vi "Register Events.vi"(8 "Error In":errorcluster, 11 "WebView in":refnum<class "WebView.lvclass">) -> (0 "Error Out":errorcluster, 2 "Events":T1, 3 "WebView out":refnum<class "WebView.lvclass">)   [LabVIEW 2024, in "WebView.lvclass"]
uses:
  WebView.lvclass
  Events--cluster.ctl
  Navigation Complete Event Data--cluster.ctl
  Source Changed Event Data--cluster.ctl
  Navigation Start Event Data--cluster.ctl
  <vilib>/sklein/WebView2/Libs/Microsoft.Web.WebView2.Core.dll
  WebView.lvclass/WebView.ctl
  callbacks/Raise Navigation Complete Event.vi
  callbacks/Raise Navigation Starting Event.vi
  callbacks/Raise Source Changed Event.vi
  callbacks/Raise Document Title Changed Event.vi
  callbacks/Raise Status Bar Text Changed Event.vi
  callbacks/Raise WebMessage Received Event.vi
  callbacks/Raise Window Close Requested Event.vi
  callbacks/Raise Dom Content Loaded Event.vi
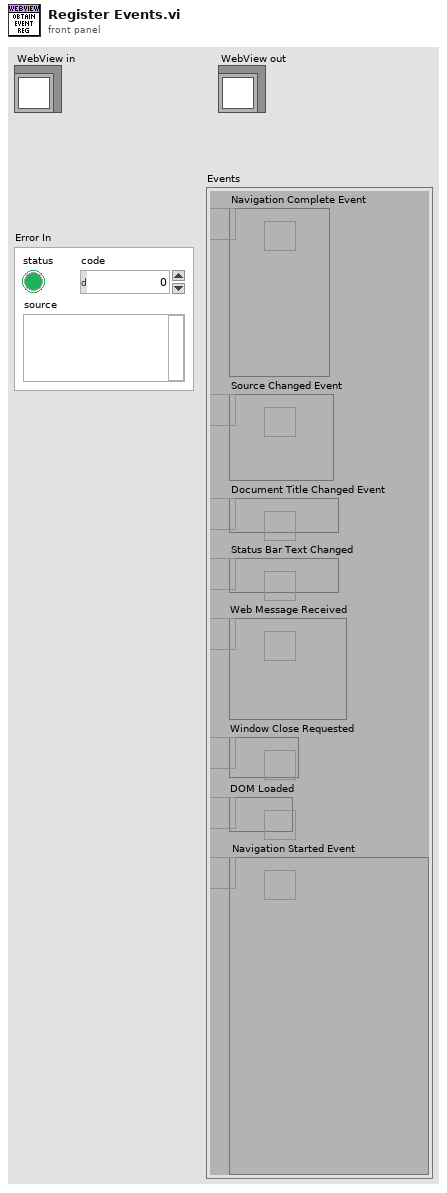
[diagram p1: front panel]
types:
  T1 = typedef "WebView.lvclass/Events--cluster.ctl" = cluster{"Navigation Complete Event":refnum<user-event>, "Source Changed Event":refnum<user-event>, "Document Title Changed Event":refnum<user-event>, "Status Bar Text Changed":refnum<user-event>, "Web Message Received":refnum<user-event>, "Window Close Requested":refnum<user-event>, "DOM Loaded":refnum<user-event>, "Navigation Started Event":refnum<user-event>}
  T2 = typedef "WebView.lvclass/Resources--cluster.ctl" = cluster{"WebView2 Control":refnum<k24>, "Webview2 Core":refnum<k24>, "event callback":refnum<k27>, "Environment":refnum<k24>}
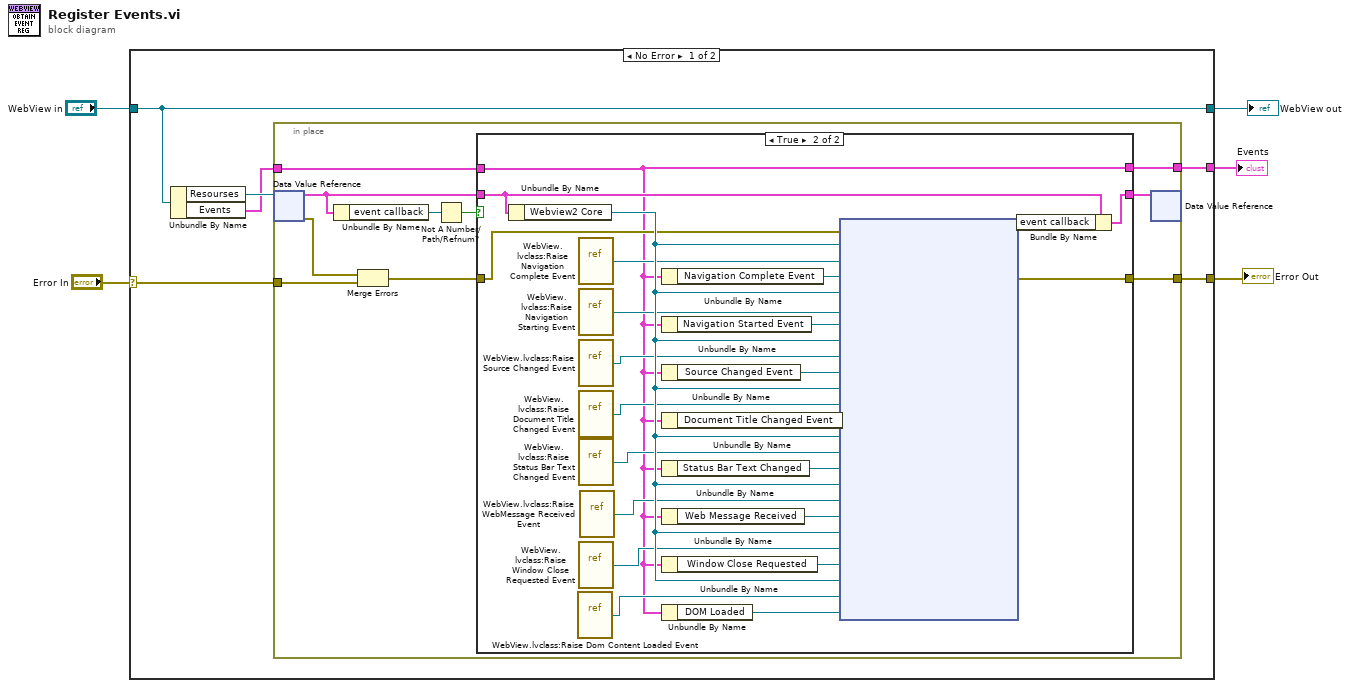
[diagram p0: block diagram]
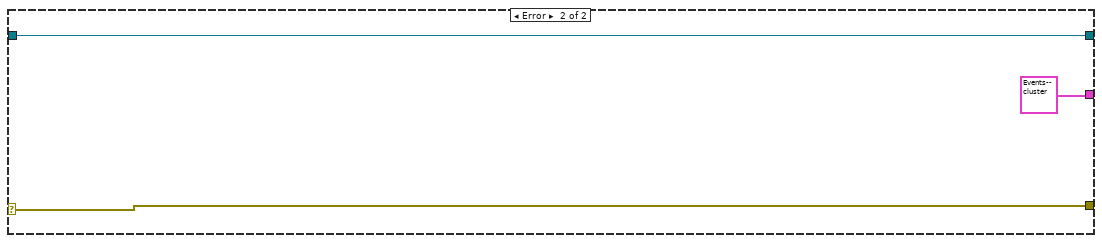
[diagram p3: hidden frame]
diagram:
  n1 = case shown="No Error" "Error In" {
    selector: "Error In" -> [w9 w50]
    tunnel: [w8 w50] -> w4
    tunnel: [w11 w49] -> w2
    tunnel: "WebView in" -> [w11 w49]
    tunnel: [w6 T1 {"Navigation Complete Event"=refnum, "Source Changed Event"=refnum, "Document Title Changed Event"=refnum, "Status Bar Text Changed"=refnum, "Web Message Received"=refnum, "Window Close Requested"=refnum, "DOM Loaded"=refnum, "Navigation Started Event"=refnum} ("Events")] -> w1
    frame No Error {
      n2 = Unbundle By Name(w11) -> ("Resourses"=w10:refnum<data-value>, "Events"=w7:T1)
      n3 = in-place {
        in-place-border: w9 -> [w21]
        in-place-border: [w18] -> w8
        in-place-border: w7 -> [w13]
        in-place-border: [w12] -> w6
        n4 = in-place-dvr #1(w10) -> (w15:T2, w20:errorcluster)
        n5 = Unbundle By Name(w15) -> ("event callback"=w17:refnum<k27>)
        n6 = Merge Errors(w20, w21) -> (w19:errorcluster)
        n7 = Not A Number/Path/Refnum?(number/path/refnum=w17) -> (NaN/Path/Refnum?=w16:bool)
        n8 = case shown="True" w16 {
          tunnel: [w24 w47] -> w18
          tunnel: w19 -> [w24 w42]
          tunnel: w15 -> [w23 w44]
          tunnel: [w23 w45] -> w14
          tunnel: w13 -> [w22 w33]
          tunnel: [w22 w33] -> w12
          frame False {
          }
          frame True {
            n9 = Unbundle By Name(w44) -> ("Webview2 Core"=w43:refnum<k24>)
            n10 = vi-ref "WebView.lvclass:Raise Dom Content Loaded Event.vi"() -> (w34:refnum<vi>)
            n11 = vi-ref "WebView.lvclass:Raise Navigation Complete Event.vi"() -> (w41:refnum<vi>)
            n12 = vi-ref "WebView.lvclass:Raise Navigation Starting Event.vi"() -> (w40:refnum<vi>)
            n13 = vi-ref "WebView.lvclass:Raise Source Changed Event.vi"() -> (w39:refnum<vi>)
            n14 = vi-ref "WebView.lvclass:Raise Document Title Changed Event.vi"() -> (w38:refnum<vi>)
            n15 = vi-ref "WebView.lvclass:Raise Status Bar Text Changed Event.vi"() -> (w37:refnum<vi>)
            n16 = vi-ref "WebView.lvclass:Raise Window Close Requested Event.vi"() -> (w35:refnum<vi>)
            n17 = vi-ref "WebView.lvclass:Raise WebMessage Received Event.vi"() -> (w36:refnum<vi>)
            n18 = Unbundle By Name(w33) -> ("Navigation Complete Event"=w32:refnum<user-event>)
            n19 = Unbundle By Name(w33) -> ("Navigation Started Event"=w31:refnum<user-event>)
            n20 = Unbundle By Name(w33) -> ("Source Changed Event"=w30:refnum<user-event>)
            n21 = Unbundle By Name(w33) -> ("Document Title Changed Event"=w29:refnum<user-event>)
            n22 = Unbundle By Name(w33) -> ("Status Bar Text Changed"=w28:refnum<user-event>)
            n23 = Unbundle By Name(w33) -> ("Web Message Received"=w27:refnum<user-event>)
            n24 = Unbundle By Name(w33) -> ("Window Close Requested"=w26:refnum<user-event>)
            n25 = Unbundle By Name(w33) -> ("DOM Loaded"=w25:refnum<user-event>)
            n26 = node(w42, w43, w41, w32, w43, w40, w31, w43, w39, w30, w43, w38, w29, w43, w37, w28, w43, w36, w27, w43, w35, w26, w43, w34, w25) -> (w46:refnum<k27>, w47:errorcluster)  [unwired: 1 in]
            n27 = Bundle By Name(cluster=w44, "event callback"=w46) -> (w45:T2)
          }
        }
        n28 = in-place-dvr #1(w14) -> ()  [unwired: 2 out]
      }
    }
    frame Error {
    }
  }
  "Error Out" <- w4
  "WebView out" <- w2
  "Events" <- w1
